vi "tripleProbeData.vi"(6 "dataCutArray":T1, 7 "tripleProbeSetting":T2={"Isat"=0, "Vfl"=0, "V+"=0, "a=1/ln2"=1.44, "Vfl*"=1.0, "[V+]*"=1.0, "Te*"=2.5, "/Rn(ohm)"=1.0, "/amplif"=1.0, "Spr, cm^2"=0.07, "plasma, a.m.u"=1.0, "Ne*10^x"=11.0} {"Ne*10^x" min=1.0 max=20.0 step=1.0; "V+" items=["14.06.17\\_0070=t0.000000-0.026000#2", "14.06.17\\_0070=t0.000000-0.026000#4", "14.06.17\\_0070=t0.000000-0.026000#6", "14.06.17\\_0071=t0.000000-0.026000#2", "14.06.17\\_0071=t0.000000-0.026000#4", "14.06.17\\_0071=t0.000000-0.026000#6", "14.06.17\\_0072=t0.000000-0.026000#2", "14.06.17\\_0072=t0.000000-0.026000#4", "14.06.17\\_0072=t0.000000-0.026000#6", "14.06.17\\_0073=t0.000000-0.026000#2", "14.06.17\\_0073=t0.000000-0.026000#4", "14.06.17\\_0073=t0.000000-0.026000#6", "14.06.17\\_0074=t0.000000-0.026000#2", "14.06.17\\_0074=t0.000000-0.026000#4", "14.06.17\\_0074=t0.000000-0.026000#6", "14.06.17\\_0075=t0.000000-0.026000#2", "14.06.17\\_0075=t0.000000-0.026000#4", "14.06.17\\_0075=t0.000000-0.026000#6", "14.06.17\\_0076=t0.000000-0.026000#2", "14.06.17\\_0076=t0.000000-0.026000#4", "14.06.17\\_0076=t0.000000-0.026000#6", "14.06.17\\_0077=t0.000000-0.026000#2", "14.06.17\\_0077=t0.000000-0.026000#4", "14.06.17\\_0077=t0.000000-0.026000#6", "14.06.17\\_0078=t0.000000-0.026000#2", "14.06.17\\_0078=t0.000000-0.026000#4", "14.06.17\\_0078=t0.000000-0.026000#6", "14.06.17\\_0079=t0.000000-0.026000#2", "14.06.17\\_0079=t0.000000-0.026000#4", "14.06.17\\_0079=t0.000000-0.026000#6", "14.06.17\\_0080=t0.000000-0.026000#2", "14.06.17\\_0080=t0.000000-0.026000#4", "14.06.17\\_0080=t0.000000-0.026000#6", "14.06.17\\_0081=t0.000000-0.026000#2", "14.06.17\\_0081=t0.000000-0.026000#4", "14.06.17\\_0081=t0.000000-0.026000#6", "14.06.17\\_0082=t0.000000-0.026000#2", "14.06.17\\_0082=t0.000000-0.026000#4", "14.06.17\\_0082=t0.000000-0.026000#6", "14.06.17\\_0083=t0.000000-0.026000#2", "14.06.17\\_0083=t0.000000-0.026000#4", "14.06.17\\_0083=t0.000000-0.026000#6", "14.06.17\\_0084=t0.000000-0.026000#2", "14.06.17\\_0084=t0.000000-0.026000#4", "14.06.17\\_0084=t0.000000-0.026000#6", "14.06.17\\_0085=t0.000000-0.026000#2", "14.06.17\\_0085=t0.000000-0.026000#4", "14.06.17\\_0085=t0.000000-0.026000#6", "14.06.17\\_0086=t0.000000-0.026000#2", "14.06.17\\_0086=t0.000000-0.026000#4", "14.06.17\\_0086=t0.000000-0.026000#6", "14.06.17\\_0086=t0.000000-0.026000#10"]; "Vfl" items=["14.06.17\\_0070=t0.000000-0.026000#2", "14.06.17\\_0070=t0.000000-0.026000#4", "14.06.17\\_0070=t0.000000-0.026000#6", "14.06.17\\_0071=t0.000000-0.026000#2", "14.06.17\\_0071=t0.000000-0.026000#4", "14.06.17\\_0071=t0.000000-0.026000#6", "14.06.17\\_0072=t0.000000-0.026000#2", "14.06.17\\_0072=t0.000000-0.026000#4", "14.06.17\\_0072=t0.000000-0.026000#6", "14.06.17\\_0073=t0.000000-0.026000#2", "14.06.17\\_0073=t0.000000-0.026000#4", "14.06.17\\_0073=t0.000000-0.026000#6", "14.06.17\\_0074=t0.000000-0.026000#2", "14.06.17\\_0074=t0.000000-0.026000#4", "14.06.17\\_0074=t0.000000-0.026000#6", "14.06.17\\_0075=t0.000000-0.026000#2", "14.06.17\\_0075=t0.000000-0.026000#4", "14.06.17\\_0075=t0.000000-0.026000#6", "14.06.17\\_0076=t0.000000-0.026000#2", "14.06.17\\_0076=t0.000000-0.026000#4", "14.06.17\\_0076=t0.000000-0.026000#6", "14.06.17\\_0077=t0.000000-0.026000#2", "14.06.17\\_0077=t0.000000-0.026000#4", "14.06.17\\_0077=t0.000000-0.026000#6", "14.06.17\\_0078=t0.000000-0.026000#2", "14.06.17\\_0078=t0.000000-0.026000#4", "14.06.17\\_0078=t0.000000-0.026000#6", "14.06.17\\_0079=t0.000000-0.026000#2", "14.06.17\\_0079=t0.000000-0.026000#4", "14.06.17\\_0079=t0.000000-0.026000#6", "14.06.17\\_0080=t0.000000-0.026000#2", "14.06.17\\_0080=t0.000000-0.026000#4", "14.06.17\\_0080=t0.000000-0.026000#6", "14.06.17\\_0081=t0.000000-0.026000#2", "14.06.17\\_0081=t0.000000-0.026000#4", "14.06.17\\_0081=t0.000000-0.026000#6", "14.06.17\\_0082=t0.000000-0.026000#2", "14.06.17\\_0082=t0.000000-0.026000#4", "14.06.17\\_0082=t0.000000-0.026000#6", "14.06.17\\_0083=t0.000000-0.026000#2", "14.06.17\\_0083=t0.000000-0.026000#4", "14.06.17\\_0083=t0.000000-0.026000#6", "14.06.17\\_0084=t0.000000-0.026000#2", "14.06.17\\_0084=t0.000000-0.026000#4", "14.06.17\\_0084=t0.000000-0.026000#6", "14.06.17\\_0085=t0.000000-0.026000#2", "14.06.17\\_0085=t0.000000-0.026000#4", "14.06.17\\_0085=t0.000000-0.026000#6", "14.06.17\\_0086=t0.000000-0.026000#2", "14.06.17\\_0086=t0.000000-0.026000#4", "14.06.17\\_0086=t0.000000-0.026000#6", "14.06.17\\_0086=t0.000000-0.026000#10"]; "Isat" items=["14.06.17\\_0070=t0.000000-0.026000#2", "14.06.17\\_0070=t0.000000-0.026000#4", "14.06.17\\_0070=t0.000000-0.026000#6", "14.06.17\\_0071=t0.000000-0.026000#2", "14.06.17\\_0071=t0.000000-0.026000#4", "14.06.17\\_0071=t0.000000-0.026000#6", "14.06.17\\_0072=t0.000000-0.026000#2", "14.06.17\\_0072=t0.000000-0.026000#4", "14.06.17\\_0072=t0.000000-0.026000#6", "14.06.17\\_0073=t0.000000-0.026000#2", "14.06.17\\_0073=t0.000000-0.026000#4", "14.06.17\\_0073=t0.000000-0.026000#6", "14.06.17\\_0074=t0.000000-0.026000#2", "14.06.17\\_0074=t0.000000-0.026000#4", "14.06.17\\_0074=t0.000000-0.026000#6", "14.06.17\\_0075=t0.000000-0.026000#2", "14.06.17\\_0075=t0.000000-0.026000#4", "14.06.17\\_0075=t0.000000-0.026000#6", "14.06.17\\_0076=t0.000000-0.026000#2", "14.06.17\\_0076=t0.000000-0.026000#4", "14.06.17\\_0076=t0.000000-0.026000#6", "14.06.17\\_0077=t0.000000-0.026000#2", "14.06.17\\_0077=t0.000000-0.026000#4", "14.06.17\\_0077=t0.000000-0.026000#6", "14.06.17\\_0078=t0.000000-0.026000#2", "14.06.17\\_0078=t0.000000-0.026000#4", "14.06.17\\_0078=t0.000000-0.026000#6", "14.06.17\\_0079=t0.000000-0.026000#2", "14.06.17\\_0079=t0.000000-0.026000#4", "14.06.17\\_0079=t0.000000-0.026000#6", "14.06.17\\_0080=t0.000000-0.026000#2", "14.06.17\\_0080=t0.000000-0.026000#4", "14.06.17\\_0080=t0.000000-0.026000#6", "14.06.17\\_0081=t0.000000-0.026000#2", "14.06.17\\_0081=t0.000000-0.026000#4", "14.06.17\\_0081=t0.000000-0.026000#6", "14.06.17\\_0082=t0.000000-0.026000#2", "14.06.17\\_0082=t0.000000-0.026000#4", "14.06.17\\_0082=t0.000000-0.026000#6", "14.06.17\\_0083=t0.000000-0.026000#2", "14.06.17\\_0083=t0.000000-0.026000#4", "14.06.17\\_0083=t0.000000-0.026000#6", "14.06.17\\_0084=t0.000000-0.026000#2", "14.06.17\\_0084=t0.000000-0.026000#4", "14.06.17\\_0084=t0.000000-0.026000#6", "14.06.17\\_0085=t0.000000-0.026000#2", "14.06.17\\_0085=t0.000000-0.026000#4", "14.06.17\\_0085=t0.000000-0.026000#6", "14.06.17\\_0086=t0.000000-0.026000#2", "14.06.17\\_0086=t0.000000-0.026000#4", "14.06.17\\_0086=t0.000000-0.026000#6", "14.06.17\\_0086=t0.000000-0.026000#10"]}) -> (3 "Array":waveform(dbl)[](array[waveform]))   [LabVIEW 2014]
panel:
  # "Te=([V+]-[Vfl])*a"
  # "Vpl=Vfl+d*Te"
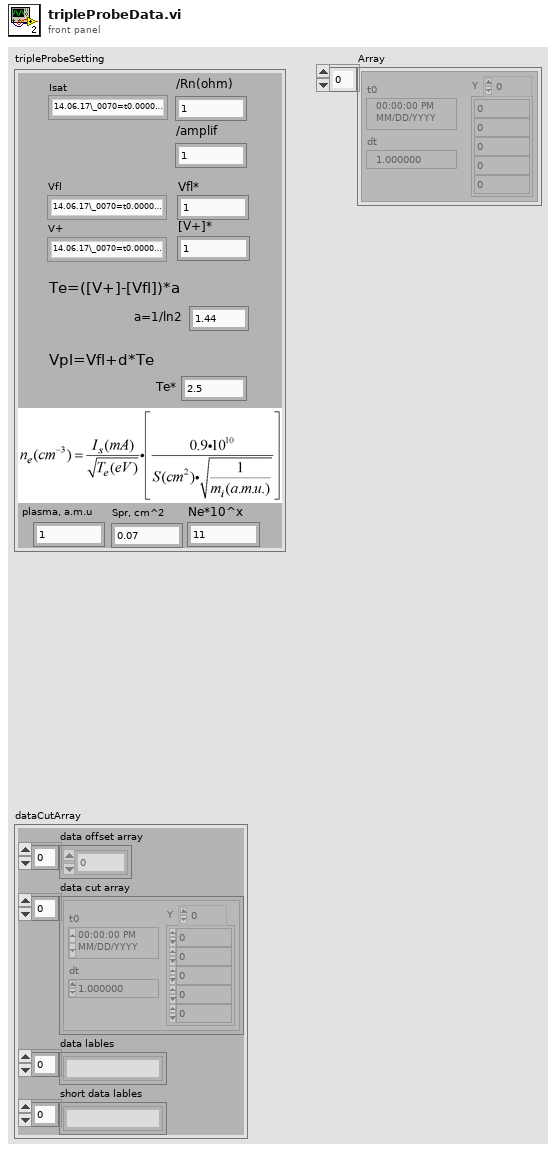
[diagram p1: front panel]
types:
  T1 = cluster{"data offset array":dbl[], "data cut array":waveform(dbl)[], "data lables":string[], "short data lables":string[]}
  T2 = cluster{"Isat":u16, "Vfl":u16, "V+":u16, "a=1/ln2":dbl, "Vfl*":dbl, "[V+]*":dbl, "Te*":dbl, "/Rn(ohm)":dbl, "/amplif":dbl, "Spr, cm^2":dbl, "plasma, a.m.u":dbl, "Ne*10^x":dbl}
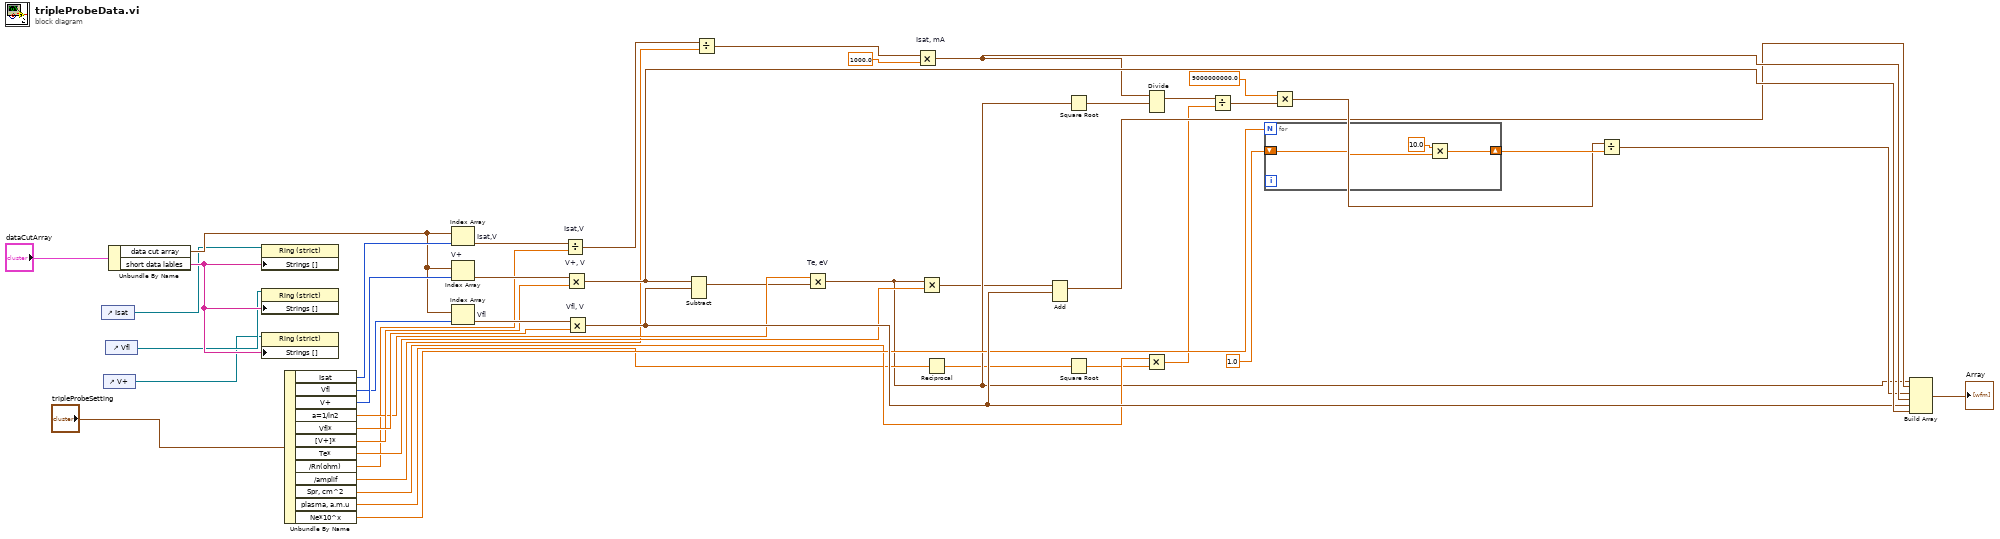
[diagram p0: block diagram]
diagram:
  n1 = control-ref of="Isat"() -> (w3:refnum<vi>)
  n2 = control-ref of="V+"() -> (w1:refnum<vi>)
  n3 = control-ref of="Vfl"() -> (w2:refnum<vi>)
  n4 = Unbundle By Name("dataCutArray") -> ("data cut array"=w5:waveform(dbl)[], "short data lables"=w6:string[])
  n5 = property on="Property Node" class="Ring (strict)"(reference=w3, "Strings []"=w6) -> ()  [unwired: 1 in, 2 out]
  n6 = property on="Property Node" class="Ring (strict)"(reference=w2, "Strings []"=w6) -> ()  [unwired: 1 in, 2 out]
  n7 = property on="Property Node" class="Ring (strict)"(reference=w1, "Strings []"=w6) -> ()  [unwired: 1 in, 2 out]
  n8 = Unbundle By Name("tripleProbeSetting") -> ("Isat"=w22:u16, "Vfl"=w23:u16, "V+"=w24:u16, "a=1/ln2"=w27:dbl, "Vfl*"=w29:dbl, "[V+]*"=w28:dbl, "Te*"=w30:dbl, "/Rn(ohm)"=w25:dbl, "/amplif"=w26:dbl, "Spr, cm^2"=w32:dbl, "plasma, a.m.u"=w31:dbl, "Ne*10^x"=w36:dbl)
  n9 = Index Array "Isat,V"(array=w5, index=w22) -> (element=w38:waveform(dbl))
  n10 = Index Array "V+"(array=w5, index=w24) -> (element=w40:waveform(dbl))
  n11 = Index Array "Vfl"(array=w5, index=w23) -> (element=w39:waveform(dbl))
  n12 = Divide "Isat,V"(x=w38, y=w25) -> (x/y=w9:waveform(dbl))
  n13 = Multiply "V+, V"(x=w40, y=w28) -> (x*y=w44:waveform(dbl))
  n14 = Multiply "Vfl, V"(x=w39, y=w29) -> (x*y=w43:waveform(dbl))
  n15 = Subtract(1:w43, 2:w44) -> (0:w7:waveform(dbl))  [unwired: 1 in, 1 out]
  n16 = Divide(x=w9, y=w26) -> (x/y=w10:waveform(dbl))
  n17 = Multiply "Te, eV"(x=w27, y=w7) -> (x*y=w19:waveform(dbl))
  n18 = Multiply "Isat, mA"(x=w10, y=1000.0) -> (x*y=w42:waveform(dbl))
  n19 = Multiply(x=w19, y=w30) -> (x*y=w8:waveform(dbl))
  n20 = Reciprocal(x=w31) -> (1/x=w12:dbl)
  n21 = Add(1:w43, 2:w8) -> (0:w20:waveform(dbl))  [unwired: 1 in, 1 out]
  n22 = Square Root(x=w19) -> (sqrt(x)=w14:waveform(dbl))
  n23 = Square Root(x=w12) -> (sqrt(x)=w13:dbl)
  n24 = Divide(1:w14, 2:w42) -> (0:w16:waveform(dbl))  [unwired: 1 in, 1 out]
  n25 = Multiply(x=w32, y=w13) -> (x*y=w15:dbl)
  n26 = Divide(x=w16, y=w15) -> (x/y=w17:waveform(dbl))
  n27 = for {
    N: w36 -> [_]
    shift-right: [w46] -> w37
    shift-left: 1.0 -> [w47]
    n28 = Multiply(x=10.0, y=w47) -> (x*y=w46:dbl)
  }
  n29 = Multiply(x=9000000000.0, y=w17) -> (x*y=w33:waveform(dbl))
  n30 = Divide(x=w33, y=w37) -> (x/y=w34:waveform(dbl))
  n31 = Build Array(w19, w20, w34, w42, w43, w44) -> (→"Array":waveform(dbl)[])
